vi "nanocal-frontend-server-18.vi"() -> ()   [LabVIEW 2018]
uses:
  nanocal/Nanocalorimetry/data/NanoCalLib.lvlibp
  publisher action.ctl
  icicle.ctl
panel:
  in  "Tab Control":enum32{"Page 1", "Page 2"}(tab)
  in  "wait (ms)":u32=20
  out "nanocal data array OUT":T1[](array[typedef])=[{"name"="frequency", "units"="Hz", "data"=59.21510317799475}, {"name"="Cs/T", "units"="J/K^2", "data"=1.24915044334812e-12}, {"name"="Ts", "units"="K", "data"=13.456821346295685}, {"name"="Cr/T", "units"="J/K^2", "data"=1.3468979938423544e-17}, {"name"="Tr", "units"="K", "data"=6.702259050679946}, {"name"="Ks", "units"="W/K", "data"=8.452345858606831e-09}, {"name"="Kr", "units"="W/K", "data"=1.5793868502253248e-14}, {"name"="Rs-therm", "units"="Ohm", "data"=4245.50086715559}, {"name"="Rr-therm", "units"="Ohm", "data"=5193.54439937376}]
  in  "Stop":bool
  # "nanocal -- frontend"
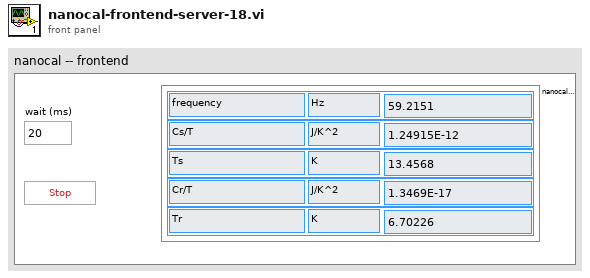
[diagram p1: front panel]
types:
  T1 = typedef "icicle.ctl" = cluster{"name":string, "units":string, "data":dbl}
  T2 = typedef "publisher action.ctl" = enum16{"set", "get", "init", "check"}
  T3 = typedef "NanoCalLib.lvlibp/NanoReadings.lvlib/NanoReadings_Parameters_TypeDef.ctl" = cluster{"Power":T4, "C and K":T5, "IV dc":T6, "Tdc,Tac":T7, "Phases":T8, "f etc":T9, "IV 1st harm":T10, "ForAveraging":cluster{"SinTherm":dbl[], "CosTherm":dbl[], "SinHeats":dbl[], "CosHeats":dbl[]}, "Output":T11, "Magnetic field etc.":T12, "Calibration":T13, "CT etc":T14, "IV 2nd harm":T15, "Resistance":T16, "Time etc":T17}
  T4 = typedef "NanoCalLib.lvlibp/NanoReadings.lvlib/NanoReadings_Power.ctl" = cluster{"PHs (W)":dbl, "PHr (W)":dbl, "Ps,dc (W)":dbl, "Pr,dc (W)":dbl, "PHs,dc (W)":dbl, "PHr,dc (W)":dbl, "Ps,ac (W)":dbl, "Pr,ac (W)":dbl, "PHs/PHr":dbl, "Poffs (W)":dbl, "Ps total (W)":dbl, "Pr total (W)":dbl, "Ps-Pr total (W)":dbl, "Ps,offs (W)":dbl}
  T5 = typedef "NanoCalLib.lvlibp/NanoReadings.lvlib/NanoReadings_CandK.ctl" = cluster{"Cs (J/K)":dbl, "Ks (W/K)":dbl, "Cr (J/K)":dbl, "Kr (W/K)":dbl, "Cdiff (J/K)":dbl, "Cs-Cr (J/K)":dbl, "Cdiff old style (J/K)":dbl, "Cr from S,diff (J/K)":dbl}
  T6 = typedef "NanoCalLib.lvlibp/NanoReadings.lvlib/NanoReadings_IandV.ctl" = cluster{"Is,dc (A)":dbl, "Ir,dc (A)":dbl, "Us,dc (V)":dbl, "Ur,dc (V)":dbl, "Udiff,dc (V)":dbl, "IHs dc (A)":dbl, "UHs dc (V)":dbl, "IHr dc (A)":dbl, "UHr dc (V)":dbl, "Uoffs dc (V)":dbl, "Ioffs dc (A)":dbl}
  T7 = typedef "NanoCalLib.lvlibp/NanoReadings.lvlib/NanoReadings_TdcTac.ctl" = cluster{"Ts (K)":dbl, "Tr (K)":dbl, "Tdiff from Rs,Rr":dbl, "Tdiff from Udiff (K)":dbl, "Ts,ac (K)":dbl, "Tr,ac (K)":dbl, "Tdiff,ac (K)":dbl, "Ts,ac driftcorr (K)":dbl, "Tr,ac driftcorr (K)":dbl, "Tr,ac from Ts,diff,ac (K)":dbl, "T target (K)":dbl}
  T8 = typedef "NanoCalLib.lvlibp/NanoReadings.lvlib/NanoReadings_Phases.ctl" = cluster{"Phi Is (deg)":dbl, "Phi Us (deg)":dbl, "Phi Ir (deg)":dbl, "Phi Ur (deg)":dbl, "Phi Udiff (deg)":dbl, "Phi IHs (deg)":dbl, "Phi UHs (deg)":dbl, "Phi IHr (deg)":dbl, "Phi UHr (deg)":dbl, "Phi R from S,diff (deg)":dbl, "Phi Is 1st (deg)":dbl, "Phi Us 1st (deg)":dbl, "Phi Ir 1st (deg)":dbl, "Phi Ur 1st (deg)":dbl, "Phi Udiff 1st (deg)":dbl, "Phi Udiff, raw (deg)":dbl}
  T9 = typedef "NanoCalLib.lvlibp/NanoReadings.lvlib/NanoReadings_Frequencies.ctl" = cluster{"f (Hz)":dbl, "f therm (Hz)":dbl, "omega (rad/s)":dbl, "Tan Phi S/diff":dbl, "Sin Phi":dbl, "Cos Phi":dbl, "f mix (Hz)":dbl, "tau (s)":dbl}
  T10 = typedef "NanoCalLib.lvlibp/NanoReadings.lvlib/NanoReadings_FirstHarmonic.ctl" = cluster{"Is,ac 1st (A)":dbl, "Ir,ac 1st (A)":dbl, "Us,ac 1st (V)":dbl, "Ur,ac 1st (V)":dbl, "Udiff,ac 1st (V)":dbl, "IHs (A)":dbl, "UHs (V)":dbl, "IHr (A)":dbl, "UHr (V)":dbl}
  T11 = typedef "NanoCalLib.lvlibp/NanoReadings.lvlib/NanoReadings_Output.ctl" = cluster{"S phase (deg)":dbl, "R phase (deg)":dbl, "Hs ac out (Vrms)":dbl, "Hr ac out (Vrms)":dbl, "S Therm dc out (V)":dbl, "R Therm dc out (V)":dbl, "S Therm ac out (Vrms)":dbl, "R Therm ac out (Vrms)":dbl, "Offset dc out (V)":dbl, "Hs dc out (V)":dbl, "Hr dc out (V)":dbl, "Offset ac out (Vrms)":dbl}
  T12 = typedef "NanoCalLib.lvlibp/NanoReadings.lvlib/NanoReadings_MagneticFieldEtc.ctl" = cluster{"H (T)":dbl, "T probe (K)":dbl, "Polar angle (deg)":dbl, "Azimuthal angle (deg)":dbl}
  T13 = typedef "NanoCalLib.lvlibp/NanoReadings.lvlib/NanoReadings_Calibration.ctl" = cluster{"1+Rs/RIs factor":dbl, "1+RIs/Rs factor":dbl, "Rs,scaled (ohm)":dbl, "Rr,scaled (ohm)":dbl, "R lead S (ohm)":dbl, "R lead R (ohm)":dbl, "|dlnR/dlnT| S":dbl, "|dlnR/dlnT| R":dbl, "dTs/dt (mK/s)":dbl, "dTr/dt (mK/s)":dbl}
  T14 = typedef "NanoCalLib.lvlibp/NanoReadings.lvlib/NanoReadings_CTetc.ctl" = cluster{"Cs/T (J/K^2)":dbl, "Cr/T (J/K^2)":dbl, "Cdiff/T (J/K^2)":dbl, "(Cs-Cr)/T (J/K^2)":dbl, "Cdiff/T old style (J/K^2)":dbl, "Cr/T from S,diff (J/K^2)":dbl, "Ts^2 (K^2)":dbl, "Tr^2 (K^2)":dbl}
  T15 = typedef "NanoCalLib.lvlibp/NanoReadings.lvlib/NanoReadings_2ndHarmonic.ctl" = cluster{"Is,ac (A)":dbl, "Ir,ac (A)":dbl, "Us,ac (V)":dbl, "Ur,ac (V)":dbl, "Udiff,ac (V)":dbl}
  T16 = typedef "NanoCalLib.lvlibp/NanoReadings.lvlib/NanoReadings_Resistance.ctl" = cluster{"RHs (ohm)":dbl, "RHr (ohm)":dbl, "Rs (ohm)":dbl, "Rr (ohm)":dbl, "RHs,dc (ohm)":dbl, "RHr,dc (ohm)":dbl, "Rs,ac (ohm)":dbl, "Rr,ac (ohm)":dbl, "Roffs (ohm)":dbl}
  T17 = typedef "NanoCalLib.lvlibp/NanoReadings.lvlib/NanoReadings_TimeEtc.ctl" = cluster{"Time (s)":dbl, "Datapoint index":dbl, "Datapoint time (s)":dbl}
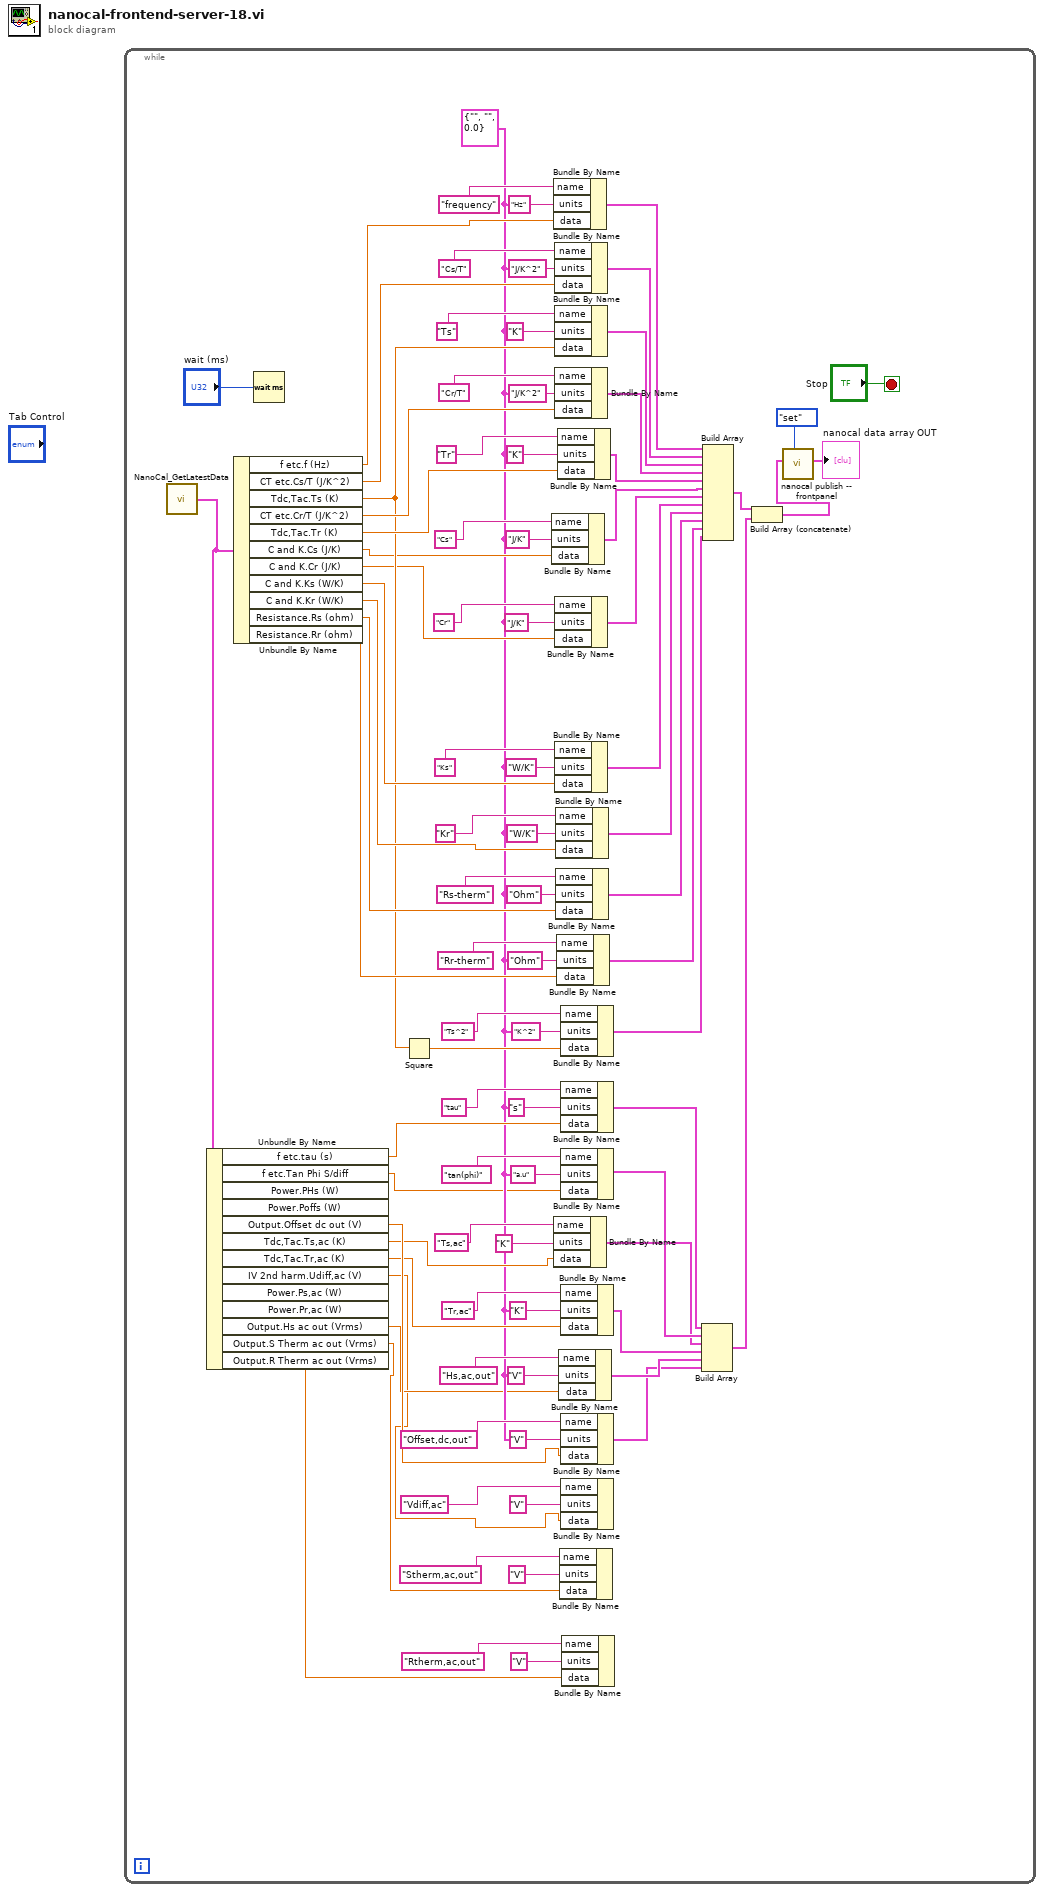
[diagram p0: block diagram]
diagram:
  n1 = while {
    stop <- "Stop" stop-if-true
    w21 = T1 {"name"="", "units"="", "data"=0.0} ("icicle")
    n2 = call "NanoCal_GetLatestData.vi"() -> ("Latest data"=w38:T3)  [unwired: 1 in]
    n3 = Unbundle By Name(w38) -> ("f etc.tau (s)"=w29:dbl, "f etc.Tan Phi S/diff"=w20:dbl, "Output.Offset dc out (V)"=w26:dbl, "Tdc,Tac.Ts,ac (K)"=w25:dbl, "Tdc,Tac.Tr,ac (K)"=w24:dbl, "IV 2nd harm.Udiff,ac (V)"=w3:dbl, "Output.Hs ac out (Vrms)"=w19:dbl, "Output.S Therm ac out (Vrms)"=w2:dbl, "Output.R Therm ac out (Vrms)"=w1:dbl)  [unwired: 4 out]
    n4 = Unbundle By Name(w38) -> ("f etc.f (Hz)"=w85:dbl, "CT etc.Cs/T (J/K^2)"=w77:dbl, "Tdc,Tac.Ts (K)"=w47:dbl, "CT etc.Cr/T (J/K^2)"=w78:dbl, "Tdc,Tac.Tr (K)"=w71:dbl, "C and K.Cs (J/K)"=w41:dbl, "C and K.Cr (J/K)"=w40:dbl, "C and K.Ks (W/K)"=w67:dbl, "C and K.Kr (W/K)"=w61:dbl, "Resistance.Rs (ohm)"=w53:dbl, "Resistance.Rr (ohm)"=w52:dbl)
    n5 = Wait (ms)(milliseconds to wait="wait (ms)") -> ()  [unwired: 1 out]
    n6 = Square(x=w47) -> (x^2=w48:dbl)
    n7 = Bundle By Name(cluster=w21, "name"="Cs", "units"="J/K", "data"=w41) -> (w44:T1)
    n8 = Bundle By Name(cluster=w21, "name"="frequency", "units"="Hz", "data"=w85) -> (w73:T1)
    n9 = Bundle By Name(cluster=w21, "name"="Ts,ac", "units"="K", "data"=w25) -> (w16:T1)
    n10 = Bundle By Name(cluster=w21, "name"="Cs/T", "units"="J/K^2", "data"=w77) -> (w74:T1)
    n11 = Bundle By Name(cluster=w21, "name"="Ts", "units"="K", "data"=w47) -> (w75:T1)
    n12 = Bundle By Name(cluster=w21, "name"="Cr/T", "units"="J/K^2", "data"=w78) -> (w76:T1)
    n13 = Bundle By Name(cluster=w21, "name"="Cr", "units"="J/K", "data"=w40) -> (w39:T1)
    n14 = Bundle By Name(cluster=w21, "name"="Ks", "units"="W/K", "data"=w67) -> (w66:T1)
    n15 = Bundle By Name(cluster=w21, "name"="Kr", "units"="W/K", "data"=w61) -> (w60:T1)
    n16 = Bundle By Name(cluster=w21, "name"="Rs-therm", "units"="Ohm", "data"=w53) -> (w55:T1)
    n17 = Bundle By Name(cluster=w21, "name"="Rr-therm", "units"="Ohm", "data"=w52) -> (w54:T1)
    n18 = Bundle By Name(cluster=w21, "name"="Tr", "units"="K", "data"=w71) -> (w70:T1)
    n19 = Bundle By Name(cluster=w21, "name"="Hs,ac,out", "units"="V", "data"=w19) -> (w14:T1)
    n20 = Bundle By Name("name"="Stherm,ac,out", "units"="V", "data"=w2) -> ()  [unwired: 1 in, 1 out]
    n21 = Bundle By Name(cluster=w21, "name"="Ts^2", "units"="K^2", "data"=w48) -> (w49:T1)
    n22 = Bundle By Name(cluster=w21, "name"="tau", "units"="s", "data"=w29) -> (w18:T1)
    n23 = Bundle By Name(cluster=w21, "name"="tan(phi)", "units"="a.u", "data"=w20) -> (w17:T1)
    n24 = Bundle By Name(cluster=w21, "name"="Tr,ac", "units"="K", "data"=w24) -> (w15:T1)
    n25 = Bundle By Name(cluster=w21, "name"="Offset,dc,out", "units"="V", "data"=w26) -> (w13:T1)
    n26 = Bundle By Name("name"="Vdiff,ac", "units"="V", "data"=w3) -> ()  [unwired: 1 in, 1 out]
    n27 = Bundle By Name("name"="Rtherm,ac,out", "units"="V", "data"=w1) -> ()  [unwired: 1 in, 1 out]
    n28 = Build Array(w18, w17, w16, w15, w14, w13) -> (w11:T1[])
    n29 = Build Array(w73, w74, w75, w76, w70, w44, w39, w66, w60, w55, w54, w49) -> (w12:T1[])
    n30 = Build Array (concatenate)(w12, w11) -> (w10:T1[])
    n31 = call "nanocal publish -- frontpanel.vi"("publisher action"=publisher_action."set", "nanocal data array IN"=w10) -> ("nanocal data array OUT"=→"nanocal data array OUT":T1[])  [unwired: 9 in]
  }
